vi "作者相关.vi"() -> ()   [LabVIEW 8.6]
panel:
  in  "?":bool
  # "个人姓名：     \n班级：07汽服\n学校：\n未婚\nQQ:\n手机："
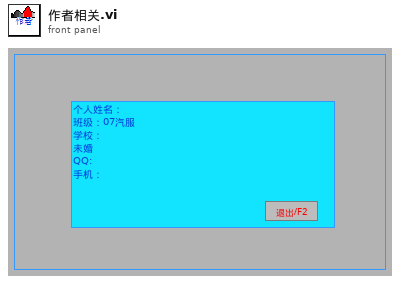
[diagram p1: front panel]
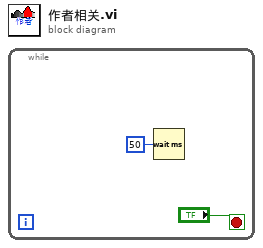
[diagram p0: block diagram]
diagram:
  n1 = while {
    stop <- "?" stop-if-true
    n2 = Wait (ms)(milliseconds to wait=u32 50 ("等待时间（毫秒）")) -> ()  [unwired: 1 out]
  }
